vi "ErrorHandling.vi"() -> ()   [LabVIEW 2012]
uses:
  <vilib>/Utility/miscctls.llb/LVPointTypeDef.ctl
  Control and Global/Global_Variables.vi
  <vilib>/Utility/error.llb/DialogType.ctl
panel:
  out "Last Error/Warning":string
  out "Error Warning History":string[][](table)
  in  "Clear Hist":bool
  in  "Show Internal Errors":bool
  out "H2 Detected":bool
  out "H2":bool
  out "N2":bool
  out "Em Stop 2":bool
  out "Em Stop Relay":bool
  out "H2 CO":bool
  out "O2":bool
  out "Air":bool
  out "USV: No 230V":bool
  out "Watch Dog":bool
  out "H2 100W":bool
  out "N2 100W":bool
  out "H2 CO 100W":bool
  out "O2 100W":bool
  out "Air 100W":bool
  out "New MesErr file to load 1kW":bool
  in  "More/Less":bool
  in  "Em Stop":bool
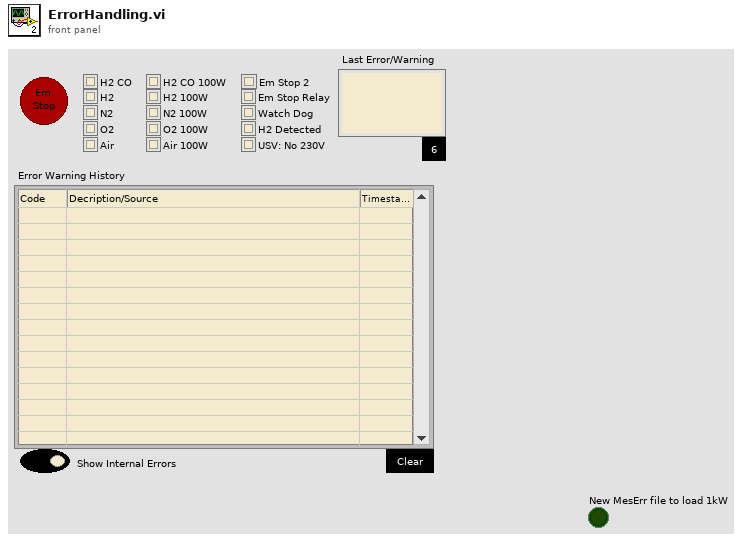
[diagram p1: front panel]
types:
  T1 = typedef "LVPointTypeDef.ctl" = cluster{"Horizontal":i16, "Vertical":i16}
  T2 = cluster{"Em. Button pressed":bool, "Em. Relay In":bool, "H2 detected":bool, "Watch Dog In":bool, "P_H2 not OK (1)":bool, "P_H2 not OK (2)":bool, "P_N2 not OK (1)":bool, "P_N2 not OK (2)":bool, "P_H2CO not OK (1)":bool, "P_H2CO not OK (2)":bool, "P_O2 not OK (1)":bool, "P_O2 not OK (2)":bool, "P_Air not OK (1)":bool, "P_Air not OK (2)":bool, "I/O 14 MUX":bool, "I/O 15 MUX":bool, "I/O 5":bool, "EM Stop Relay Out":bool, "Watch Dog Out":bool, "USV: No ~230V":bool}
  T3 = cluster{"f1":bool, "f2":bool, "f2":bool, "f3":bool, "New MesErr file to load":bool, "New Command file to load":bool, "f6":bool, "f7":bool, "New MesErr file to load 100W":bool, "New Command file to load 100W":bool}
  T4 = cluster{"Internal Error 1kW":bool, "Test Error 1kW":bool, "Shut down test":bool, "Terminate programm":bool, "Set secure state":bool, "Test is running":bool, "Flush after Error 1kW":bool, "f07":bool, "f08":bool, "Command file created":bool, "f10":bool, "f11":bool, "f12":bool, "f13":bool, "Logging":bool, "Is Measuring Cell Imp.":bool, "Test is running 100W":bool, "Command file created 100W":bool, "Shut down test 100W":bool, "Logging 100W":bool, "Internal Error 100W":bool, "Test Error 100W":bool, "Internal Error":bool, "Set secure state 100W":bool, "Flush after Error 100W":bool, "Init_Dnet":bool, "Use Stopsequenz 1kW":bool, "Use Stopsequenz 100W":bool, "Do Stopsequenz 1kW":bool, "Do Stopsequenz 100W":bool}
  T5 = typedef "Semaphore RefNum" = refnum<k1>
  T6 = typedef "DialogType.ctl" = u16
  T7 = typedef "TB1kW_Controls.lvlib/Format_Error.ctl" = cluster{"Name":string, "Options":dbl[], "Last check at:":timestamp}
  T8 = typedef "TB1kW_Controls.lvlib/Test_Properties.ctl" = cluster{"Cell Properties":T9, "Time":T10, "Flow N2 to Ox [Nl/min]":dbl, "Flow N2 to Fuel [Nl/min]":dbl, "Flush time after test error [s]":dbl, "Used Gases":cluster{"H2":bool, "N2":bool, "Air":bool, "O2":bool, "CO H2":bool}, "Fuelcell Temp. [°C]":dbl, "CO mixing ratio in tank [ppm]":dbl, "Stoichiometry Fuel [-]":dbl, "N2 in Fuel [%]":dbl, "Stoichiometry Ox [-]":dbl, "CO in Fuel [ppm]":dbl, "Humidity Ox [%]":dbl, "Humidity Fuel [%]":dbl, "Making I/U Curve":bool, "Meas Cell Impedance":bool, "Imped. Meas Intervall [s]":u32, "Nr. of Comand-Files Rep.":u32, "Use PS1":bool, "Use PS2":bool, "Use cyrostat":bool, "Used Temp Sens":cluster{"Temp 0":bool, "Temp 1":bool, "Temp 2":bool, "Temp 3":bool, "Temp 4":bool, "Temp 5":bool, "Temp 6":bool, "Temp 7":bool}, "Adjust AIn":cluster{"Gain":dbl, "Zero":dbl, "Unit":string}[]}
  T9 = typedef "TB1kW_Controls.lvlib/Cell_Properties.ctl" = cluster{"Nr of cells [-]":u8, "Cell area [cm2]":dbl, "Min. stack voltage [V]":dbl, "Min. cell voltage [mV]":dbl, "Max. stack current [A]":dbl, "Max. Dcell voltage [mV]":dbl, "Last Cell on Pin":i8, "First Cell on Pin":i8}
  T10 = typedef "TB1kW_Controls.lvlib/Time.ctl" = cluster{"[hh:mm:ss]\n[DD/MM/YY]":timestamp, "Include date":bool, "Time used as":string, "[hh:mm:ss]":dbl}
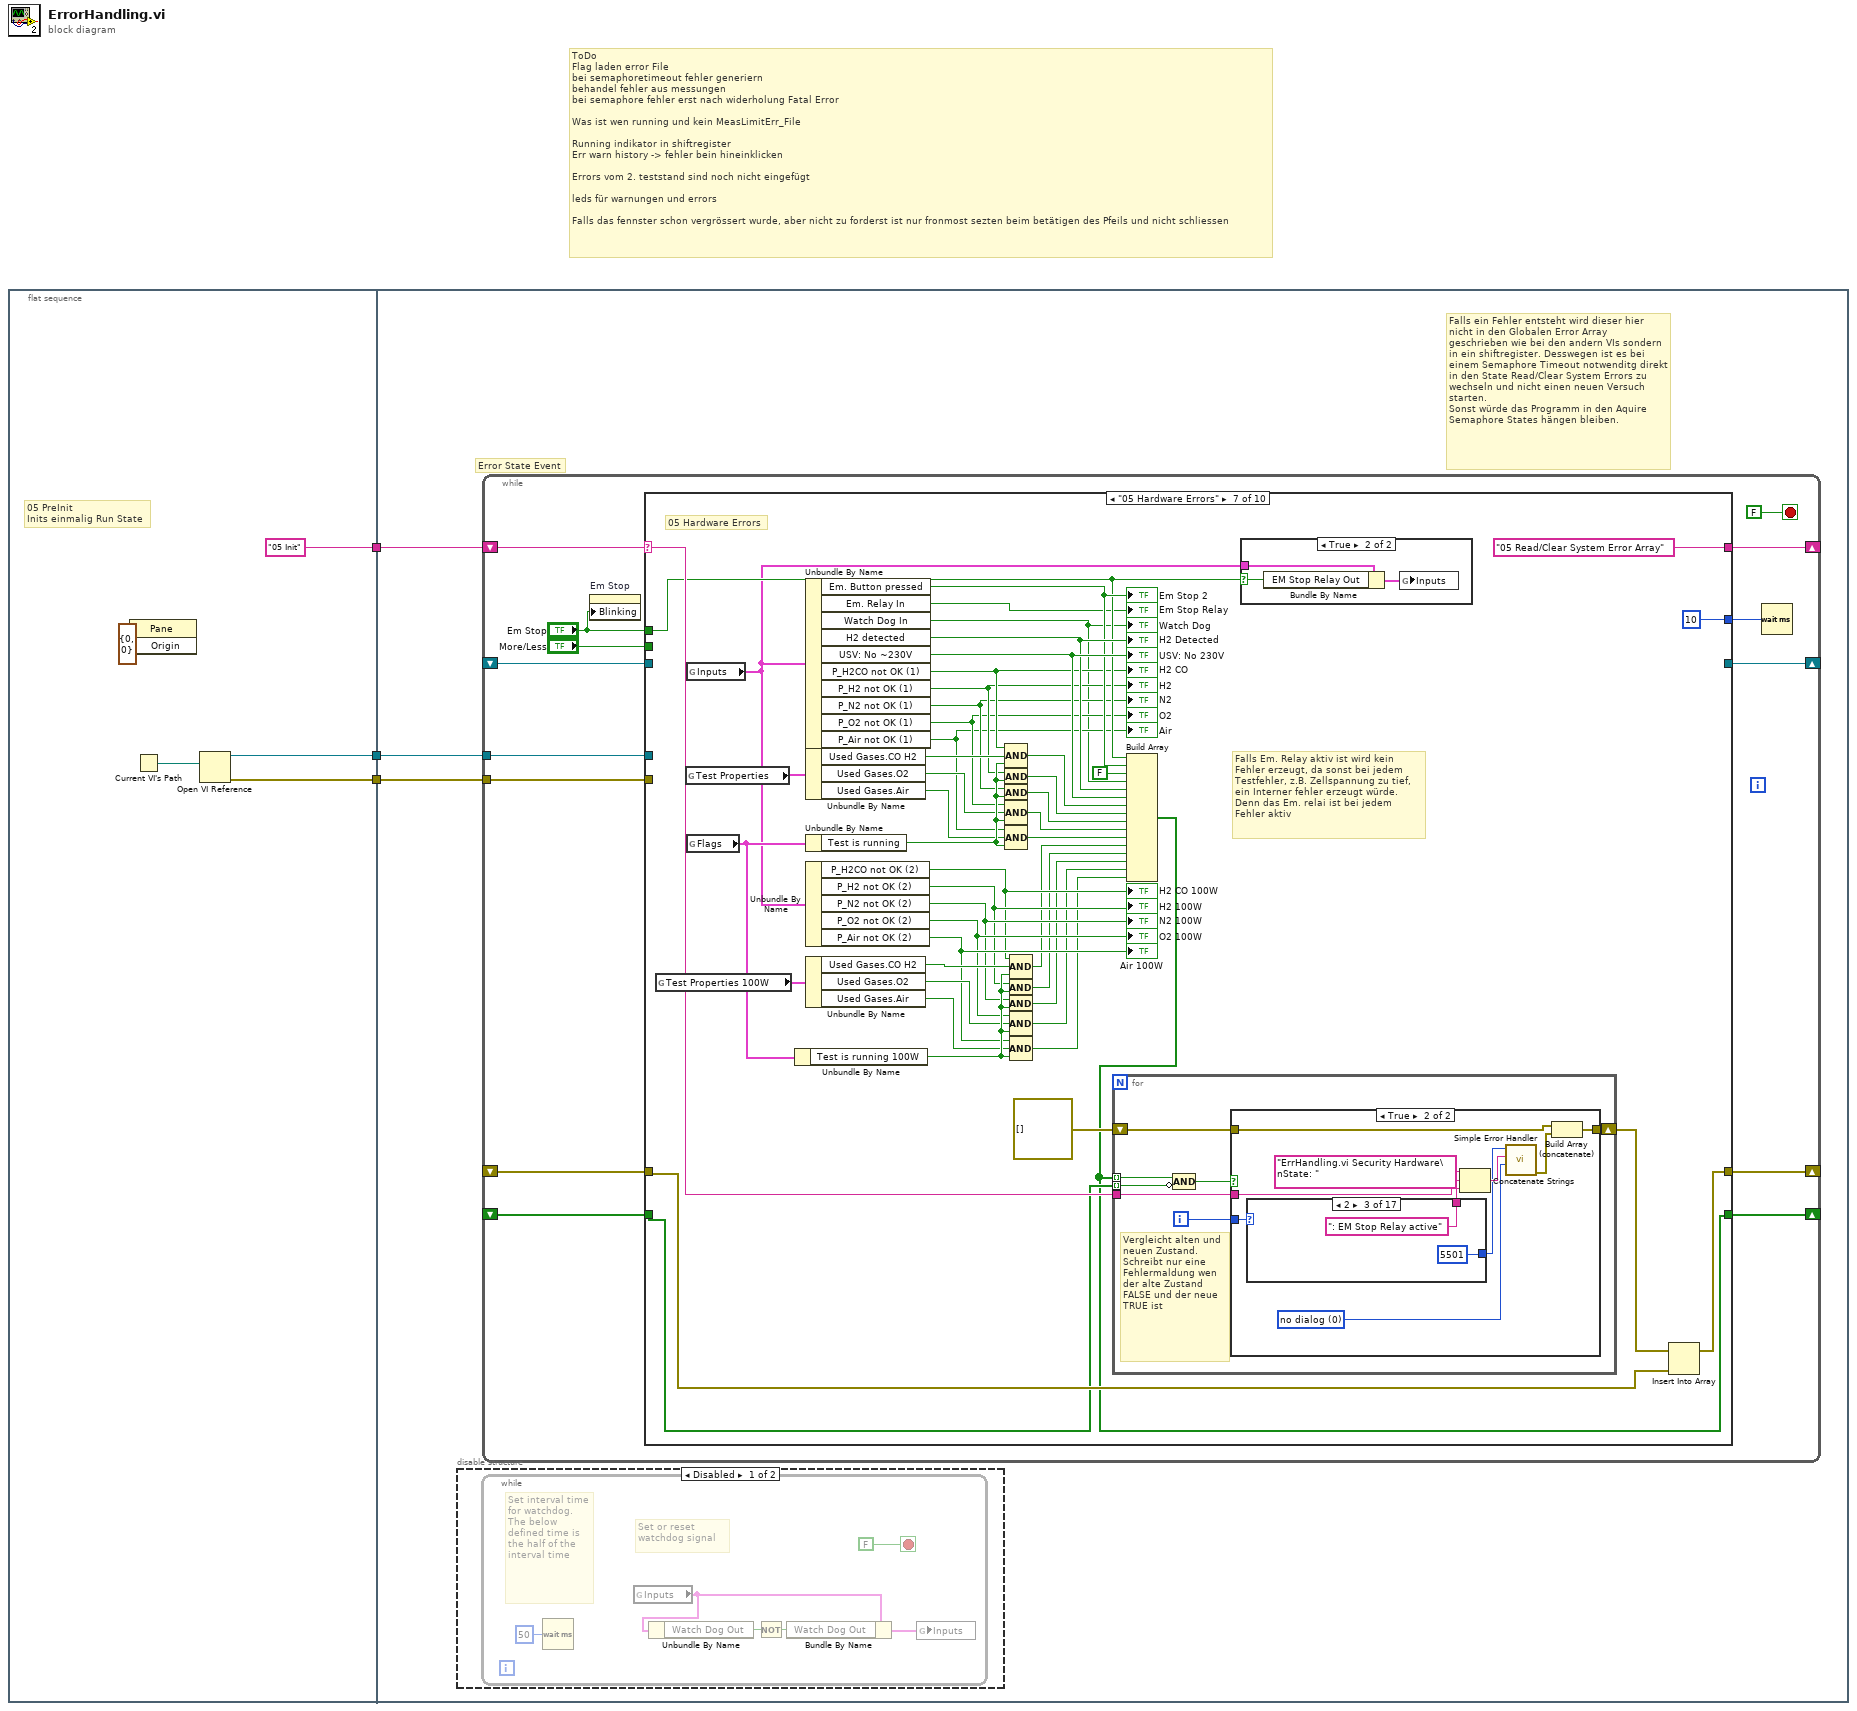
[diagram p0: block diagram]
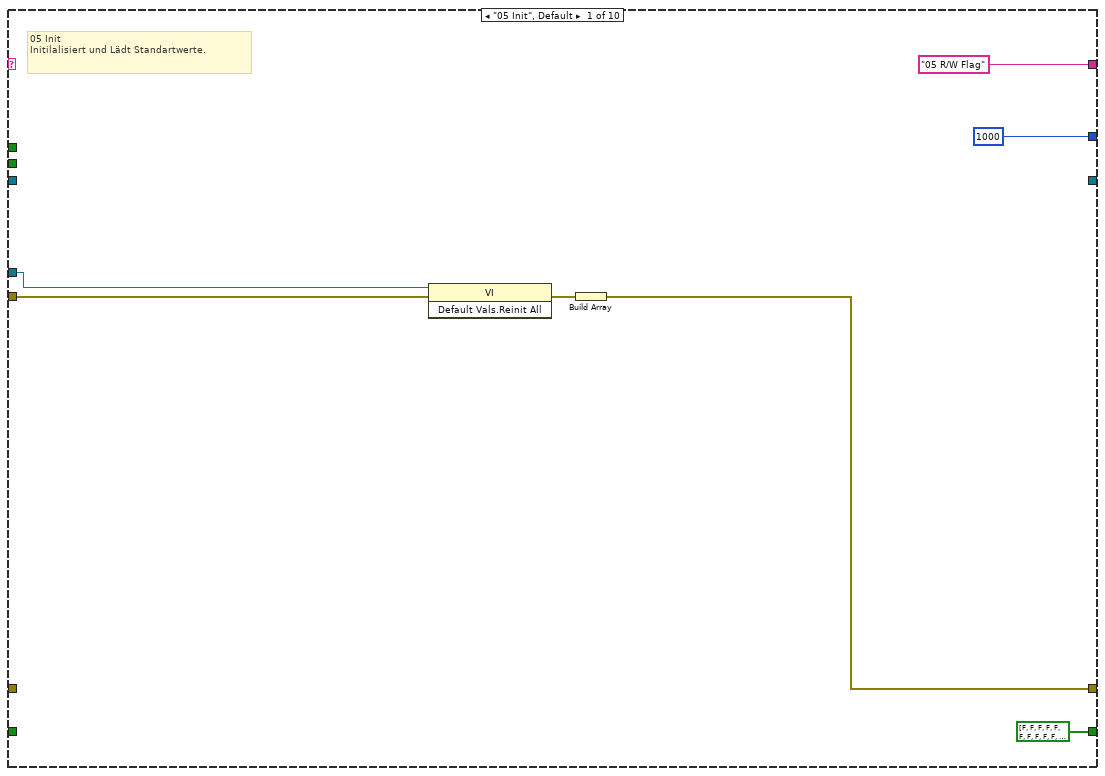
[diagram p3: hidden frame]
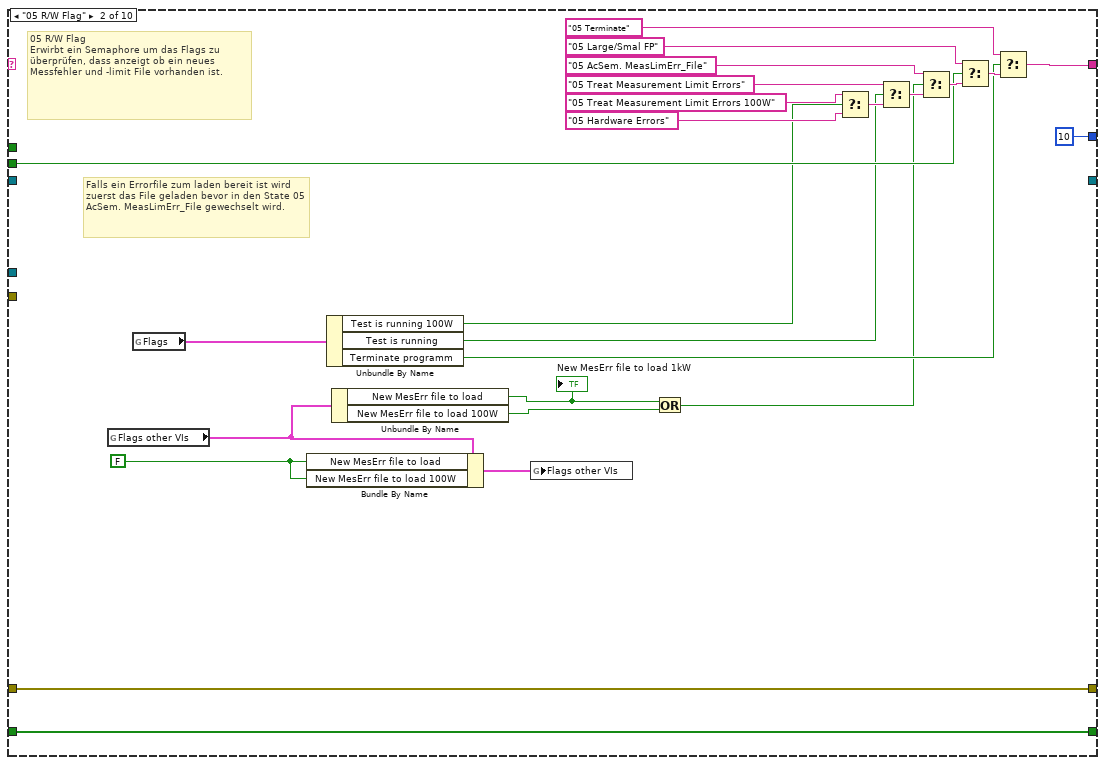
[diagram p4: hidden frame]
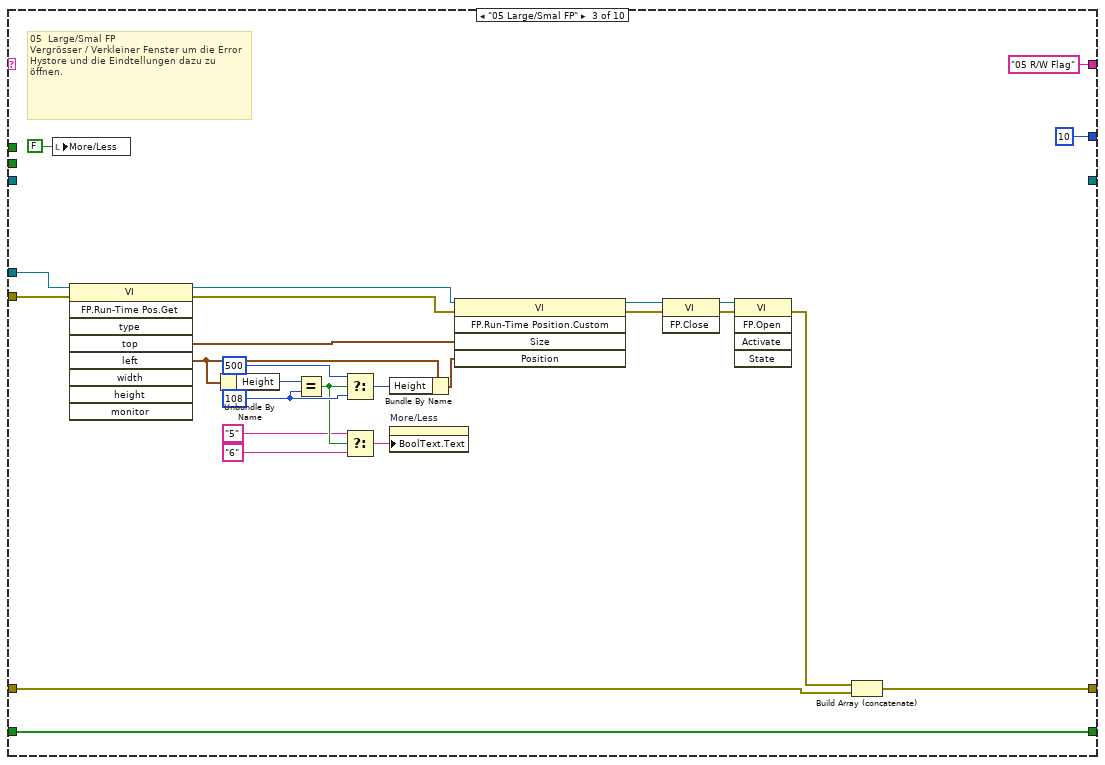
[diagram p5: hidden frame]
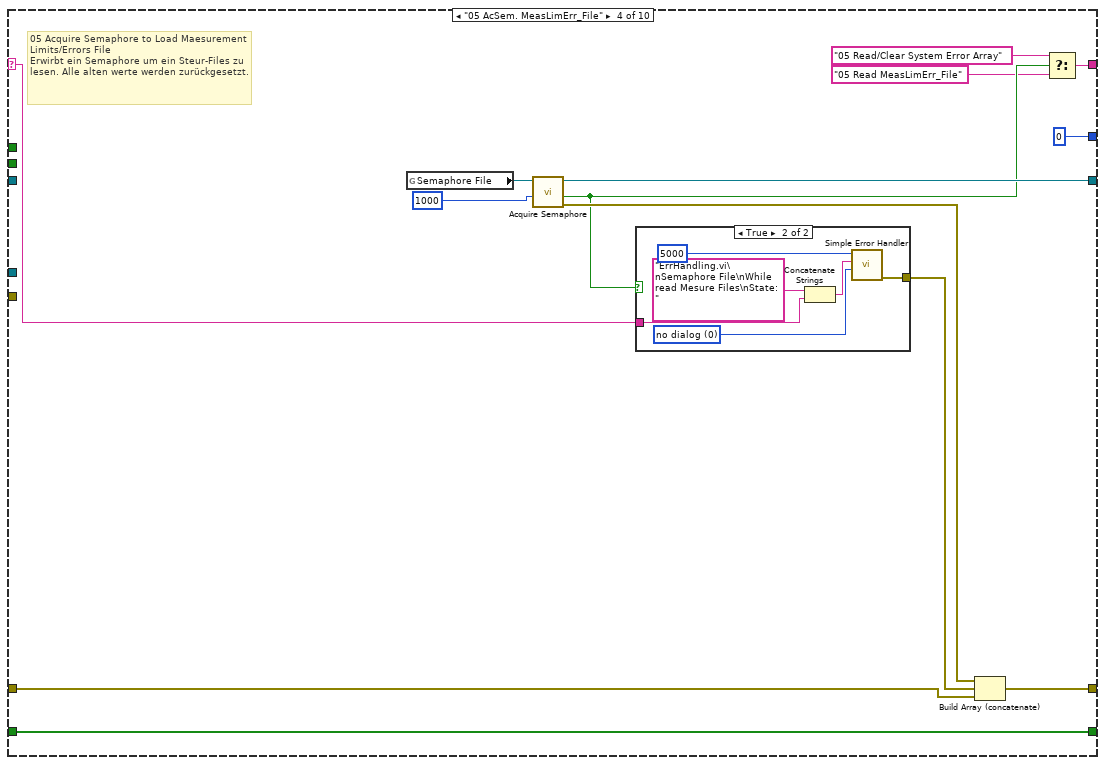
[diagram p6: hidden frame]
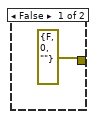
[diagram p7: hidden frame]
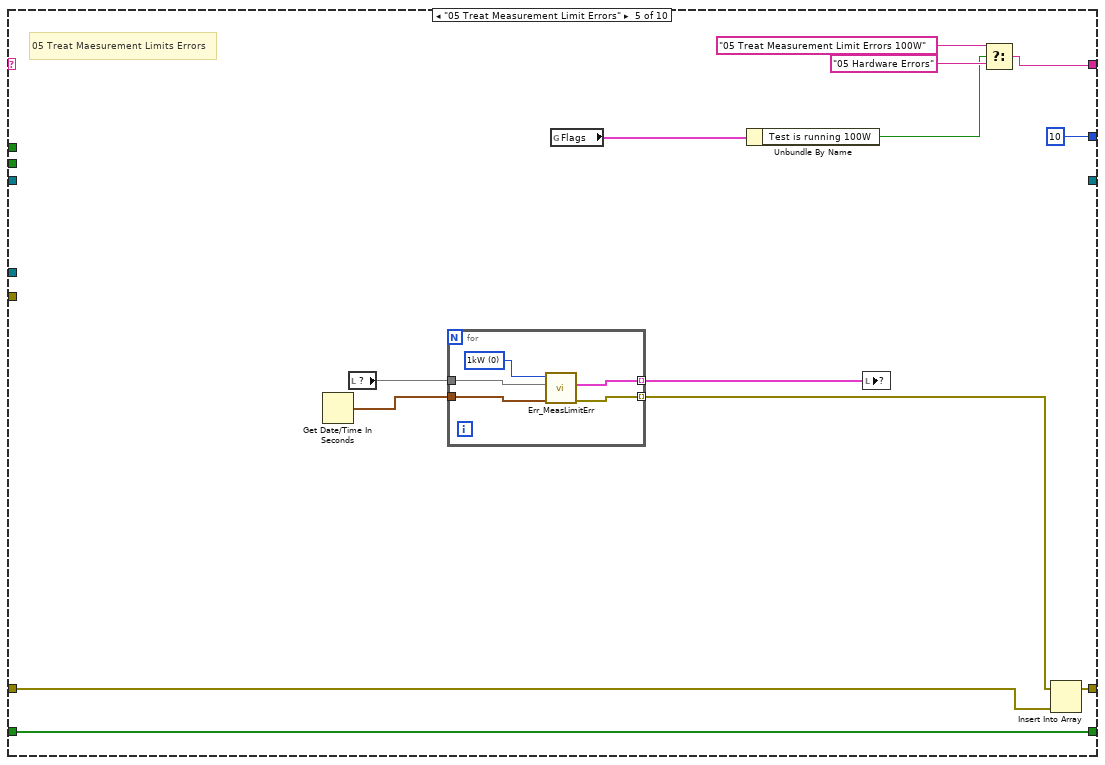
[diagram p8: hidden frame]
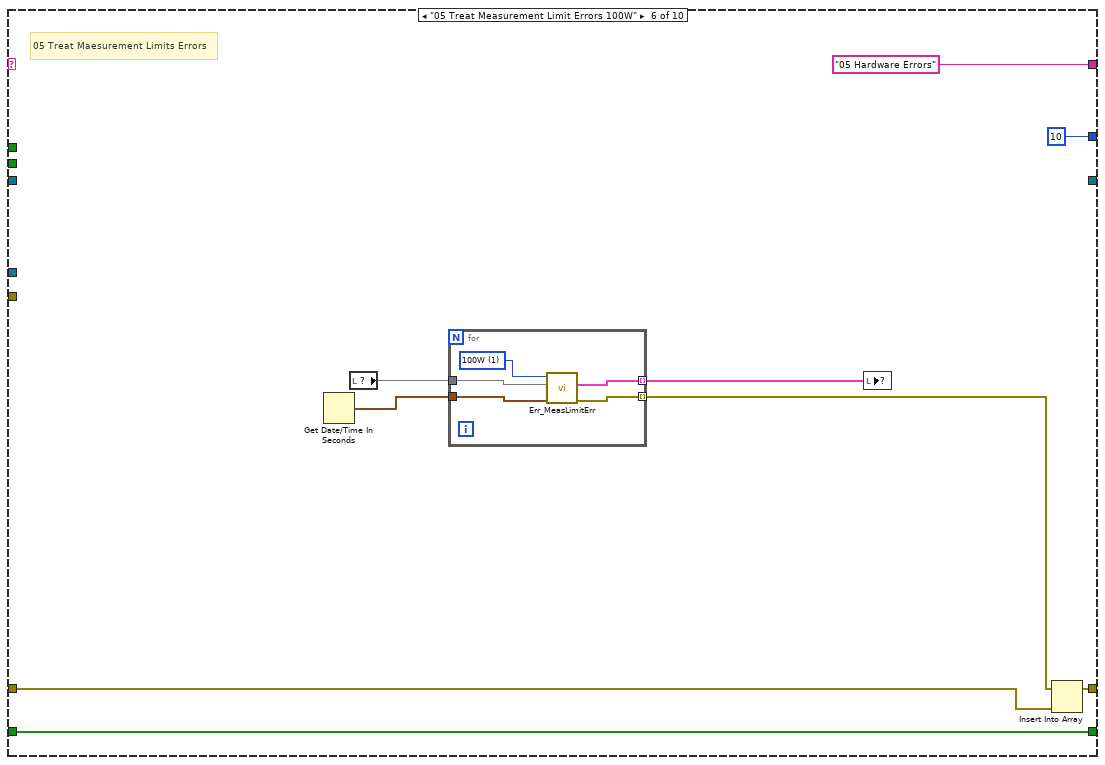
[diagram p9: hidden frame]
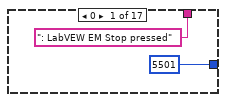
[diagram p12: hidden frame]
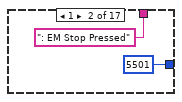
[diagram p13: hidden frame]
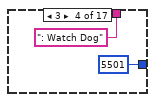
[diagram p14: hidden frame]
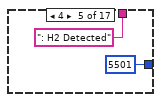
[diagram p15: hidden frame]
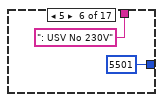
[diagram p16: hidden frame]
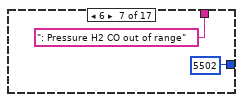
[diagram p17: hidden frame]
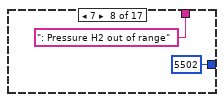
[diagram p18: hidden frame]
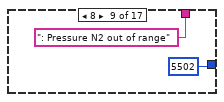
[diagram p19: hidden frame]
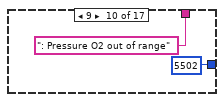
[diagram p20: hidden frame]
diagram:
  # "ToDo\nFlag laden error File\nbei semaphoretimeout fehler generiern\nbehandel fehler aus messungen\nbei semaphore fehler erst nach widerholung Fatal Error\n\nWas ist wen running und kein MeasLimitErr_File\n\nRunning indikator in shiftregister\nErr warn history -> fehler bein hineinklicken\n\nErrors vom 2. teststand sind noch nicht eingefügt\n\nleds für warnungen und errors\n\nFalls das fennster schon vergrössert wurde, aber nicht zu forderst ist nur fronmost sezten beim betätigen des Pfeils und nicht schliessen"
  n1 = flat-sequence {
    tunnel: [w8] -> w3
    tunnel: [w7] -> w2
    tunnel: ["05 Init" ("name or relative path")] -> w1
    tunnel: w3 -> [w11]
    tunnel: w2 -> [w10]
    tunnel: w1 -> [w9]
    frame #0 {
      # "05 PreInit\nInits einmalig Run State"
      n2 = property on="Property Node" class="Pane"("Origin"=T1 {"Horizontal"=0, "Vertical"=0}) -> ()  [unwired: 2 in, 2 out]
      n3 = Current VI's Path() -> (path=w6:path)
      n4 = Open VI Reference(vi path=w6) -> (vi reference=w8:refnum<vi>, error out=w7:errorcluster)  [unwired: 2 in, 3 out]
    }
    frame #1 {
      # "Falls ein Fehler entsteht wird dieser hier nicht in den Globalen Error Array geschrieben wie bei den andern VIs sondern in ein shiftregister. Desswegen ist es bei einem Semaphore Timeout notwenditg direkt in den State Read/Clear System Errors zu wechseln und nicht einen neuen Versuch starten.\nSonst würde das Programm in den Aquire Semaphore States hängen bleiben."
      # "Error State Event"
      n5 = disable-structure shown="Disabled" {
        frame Disabled {
          n6 = while {
            stop <- FALSE stop-if-true
            # "Set interval time for watchdog. The below defined time is the half of the interval time"
            # "Set or reset watchdog signal"
            n7 = Wait (ms)(milliseconds to wait=u32 50 ("Zu wartende ms")) -> ()  [unwired: 1 out]
            n8 = global read "Global_Variables.vi" "Inputs"() -> (w13:T2)
            n9 = Unbundle By Name(w13) -> ("Watch Dog Out"=w15:bool)
            n10 = Not(x=w15) -> (.not. x?=w16:bool)
            n11 = Bundle By Name(cluster=w13, "Watch Dog Out"=w16) -> (w14:T2)
            n12 = global write "Global_Variables.vi" "Inputs"(w14) -> ()
          }
        }
        frame Enabled {
        }
      }
      n13 = while {
        shift-right: [w24] -> _
        shift-left: w9 -> [w22]
        shift-right: [w29] -> _
        shift-left: _ -> [w28]
        tunnel: w11 -> [w27]
        tunnel: w10 -> [w26]
        shift-right: [w30] -> _
        shift-left: _ -> [w25]
        shift-right: [w20] -> _
        shift-left: _ -> [w19]
        stop <- FALSE stop-if-true
        n14 = property on="Em Stop" class="Bool (strict)"("Blinking"="Em Stop") -> ()  [unwired: 2 in, 2 out]
        n15 = case shown="\"05 Hardware Errors\"" w22 {
          selector: w22 -> [_ _ _ w97 _ _ w188 _ _ _]
          tunnel: ["05 R/W Flag" w50 "05 R/W Flag" w103 w111 "05 Hardware Errors" "05 Read/Clear System Error Array" "05 Treat All Errors" "05 R/W Flag" "05 Terminate"] -> w24
          tunnel: [u32 1000 ("milliseconds to wait") u32 10 ("milliseconds to wait") u32 10 ("milliseconds to wait") u32 0 ("milliseconds to wait") u32 10 ("milliseconds to wait") u32 10 ("milliseconds to wait") u32 10 ("milliseconds to wait") u32 10 ("milliseconds to wait") u32 10 ("milliseconds to wait") u32 10 ("milliseconds to wait")] -> w23
          tunnel: w28 -> [_ _ _ _ _ _ _ _ _ _]
          tunnel: w27 -> [w35 _ w80 _ _ _ _ _ _ w338]
          tunnel: w26 -> [w36 _ w79 _ _ _ _ _ _ w337]
          tunnel: [_ _ _ w96 _ _ _ _ _ _] -> w29
          tunnel: [w34 w61 w82 w93 w118 w132 w161 w248 errorcluster[] [] w334] -> w30
          tunnel: w25 -> [_ w61 w83 w94 w119 w131 w163 w249 w260 w333]
          tunnel: "More/Less" -> [_ w54 _ _ _ _ _ _ _ _]
          tunnel: "Em Stop" -> [_ _ _ _ _ _ w175 _ _ _]
          tunnel: [bool[] [FALSE, FALSE, FALSE, FALSE, FALSE, FALSE, FALSE, FALSE, FALSE, FALSE, FALSE, FALSE, FALSE, FALSE, FALSE, FALSE, FALSE, FALSE, FALSE, FALSE, FALSE] w52 w64 w90 w116 w133 w143 w246 w257 w331] -> w20
          tunnel: w19 -> [_ w52 w64 w90 w116 w133 w162 w246 w257 w331]
          frame "05 Init", Default {
            # "05 Init\nInitilalisiert und Lädt Standartwerte."
            n16 = invoke class="VI" method="Default Vals.Reinit All"(reference=w35, error in=w36) -> (error out=w37:errorcluster)  [unwired: 1 in, 2 out]
            n17 = Build Array(w37) -> (w34:errorcluster[])
          }
          frame "05 R/W Flag" {
            w44 = FALSE ("Measurement error file created")
            # "Falls ein Errorfile zum laden bereit ist wird zuerst das File geladen bevor in den State 05 AcSem. MeasLimErr_File gewechselt wird."
            # "05 R/W Flag\nErwirbt ein Semaphore um das Flags zu überprüfen, dass anzeigt ob ein neues Messfehler und -limit File vorhanden ist."
            n18 = global read "Global_Variables.vi" "Flags other VIs"() -> (w59:T3)
            n19 = global read "Global_Variables.vi" "Flags"() -> (w60:T4)
            n20 = Bundle By Name(cluster=w59, "New MesErr file to load"=w44, "New MesErr file to load 100W"=w44) -> (w58:T3)
            n21 = Unbundle By Name(w60) -> ("Test is running 100W"=w40:bool, "Test is running"=w39:bool, "Terminate programm"=w48:bool)
            n22 = Unbundle By Name(w59) -> ("New MesErr file to load"=w47:bool, "New MesErr file to load 100W"=w46:bool)
            "New MesErr file to load 1kW" <- w47
            n23 = global write "Global_Variables.vi" "Flags other VIs"(w58) -> ()
            n24 = Or(x=w47, y=w46) -> (x .or. y?=w45:bool)
            n25 = Select(t="05 Treat Measurement Limit Errors 100W", s=w40, f="05 Hardware Errors") -> (s? t:f=w43:string)
            n26 = Select(t="05 Treat Measurement Limit Errors", s=w39, f=w43) -> (s? t:f=w62:string)
            n27 = Select(t="05 AcSem. MeasLimErr_File", s=w45, f=w62) -> (s? t:f=w55:string)
            n28 = Select(t="05 Large/Smal FP", s=w54, f=w55) -> (s? t:f=w49:string)
            n29 = Select(t="05 Terminate", s=w48, f=w49) -> (s? t:f=w50:string)
          }
          frame "05 Large/Smal FP" {
            w86 = i16 108 ("y")
            # "05  Large/Smal FP\nVergrösser / Verkleiner Fenster um die Error Hystore und die Eindtellungen dazu zu öffnen."
            n30 = local write "More/Less"(FALSE ("More/Less")) -> ()
            n31 = invoke class="VI" method="FP.Run-Time Pos.Get"(reference=w80, error in=w79) -> (reference out=w77:refnum<vi>, error out=w76:errorcluster, "top"=w74:cluster{"Top":i16, "Left":i16}, "left"=w78:cluster{"Height":i16, "Width":i16})  [unwired: 7 in, 5 out]
            n32 = Unbundle By Name(w78) -> ("Height"=w87:i16)
            n33 = Equal?(x=w87, y=w86) -> (x = y?=w68:bool)
            n34 = Select(t=i16 500 ("y"), s=w68, f=w86) -> (s? t:f=w84:i16)
            n35 = Select(t="5", s=w68, f="6") -> (s? t:f=w65:string)
            n36 = Bundle By Name(cluster=w78, "Height"=w84) -> (w75:cluster{"Height":i16, "Width":i16})
            n37 = property on="More/Less" class="Bool (strict)"("BoolText.Text"=w65) -> ()  [unwired: 2 in, 2 out]
            n38 = invoke class="VI" method="FP.Run-Time Position.Custom"(reference=w77, error in=w76, "Size"=w74, "Position"=w75) -> (reference out=w72:refnum<vi>, error out=w71:errorcluster)  [unwired: 1 in, 3 out]
            n39 = invoke class="VI" method="FP.Close"(reference=w72, error in=w71) -> (reference out=w69:refnum<vi>, error out=w70:errorcluster)  [unwired: 1 in, 1 out]
            n40 = invoke class="VI" method="FP.Open"(reference=w69, error in=w70) -> (error out=w73:errorcluster)  [unwired: 3 in, 4 out]
            n41 = Build Array (concatenate)(w73, w83) -> (w82:errorcluster[])
          }
          frame "05 AcSem. MeasLimErr_File" {
            # "05 Acquire Semaphore to Load Maesurement Limits/Errors File\nErwirbt ein Semaphore um ein Steur-Files zu lesen. Alle alten werte werden zurückgesetzt."
            n42 = global read "Global_Variables.vi" "Semaphore File"() -> (w100:T5)
            n43 = call <vilib>:"Acquire Semaphore.vi"("ms timeout (-1)"=1000, "semaphore"=w100) -> ("error out"=w99:errorcluster, "timed out"=w95:bool, "semaphore out"=w96:T5)  [unwired: 1 in, 2 out]
            n44 = case shown="True" w95 {
              tunnel: [errorcluster {"status"=FALSE, "code"=0, "source"=""} ("error out") w108] -> w98
              tunnel: w97 -> [_ w105]
              frame False {
              }
              frame True {
                w109 = T6 0 items=["no dialog", "OK message", "continue or stop message", "OK message + warnings", "continue/stop + warnings"] ("type of dialog (OK msg:1)")
                n45 = Concatenate Strings("ErrHandling.vi\nSemaphore File\nWhile read Mesure Files\nState: " ("error source (\" \")"), w105) -> (w106:string)
                n46 = call <vilib>:"Simple Error Handler.vi"("error code (no error:0)"=5000, "error source (\" \")"=w106, "type of dialog (OK msg:1)"=w109) -> ("error out"=w108:errorcluster)  [unwired: 1 in, 5 out]
              }
            }
            n47 = Build Array (concatenate)(w99, w98, w94) -> (w93:errorcluster[])
            n48 = Select(t="05 Read/Clear System Error Array", s=w95, f="05 Read MeasLimErr_File") -> (s? t:f=w103:string)
          }
          frame "05 Treat Measurement Limit Errors" {
            # "05 Treat Maesurement Limits Errors"
            n49 = Get Date/Time In Seconds() -> (seconds since 1Jan1904=w117:timestamp)
            n50 = local read item#-1() -> (w122)
            n51 = for {
              tunnel: w122 -> [w126]
              tunnel: [w128] -> w121 mode=indexing
              tunnel: [w127] -> w120 mode=indexing
              tunnel: w117 -> [w125]
              w124 = u8 0 items=["1kW", "100W"] ("Testbench")
              n52 = call "Err_MeasLimitErr.vi"("Current time"=w125, "Measurement Error Limit In"=w126, "Testbench"=w124) -> ("Error out"=w127:errorcluster, "Measurement Error Limit Out"=w128:T7)  [unwired: 3 out]
            }
            n53 = global read "Global_Variables.vi" "Flags"() -> (w115:T4)
            n54 = Unbundle By Name(w115) -> ("Test is running 100W"=w112:bool)
            n55 = local write item#-1(w121) -> ()
            n56 = Select(t="05 Treat Measurement Limit Errors 100W", s=w112, f="05 Hardware Errors") -> (s? t:f=w111:string)
            n57 = Insert Into Array(array=w120, new element=w119) -> (w118:errorcluster[])  [unwired: 1 in]
          }
          frame "05 Treat Measurement Limit Errors 100W" {
            # "05 Treat Maesurement Limits Errors"
            n58 = Get Date/Time In Seconds() -> (seconds since 1Jan1904=w134:timestamp)
            n59 = local read item#-1() -> (w137)
            n60 = for {
              tunnel: w137 -> [w140]
              tunnel: [w142] -> w136 mode=indexing
              tunnel: [w141] -> w135 mode=indexing
              tunnel: w134 -> [w139]
              w138 = u8 1 items=["1kW", "100W"] ("Testbench")
              n61 = call "Err_MeasLimitErr.vi"("Current time"=w139, "Measurement Error Limit In"=w140, "Testbench"=w138) -> ("Error out"=w141:errorcluster, "Measurement Error Limit Out"=w142:T7)  [unwired: 3 out]
            }
            n62 = local write item#-1(w136) -> ()
            n63 = Insert Into Array(array=w135, new element=w131) -> (w132:errorcluster[])  [unwired: 1 in]
          }
          frame "05 Hardware Errors" {
            # "Falls Em. Relay aktiv ist wird kein Fehler erzeugt, da sonst bei jedem Testfehler, z.B. Zellspannung zu tief, ein Interner fehler erzeugt würde. Denn das Em. relai ist bei jedem Fehler aktiv"
            # "05 Hardware Errors"
            n64 = global read "Global_Variables.vi" "Test Properties 100W"() -> (w160:T8)
            n65 = global read "Global_Variables.vi" "Test Properties"() -> (w183:T8)
            n66 = global read "Global_Variables.vi" "Inputs"() -> (w144:T2)
            n67 = global read "Global_Variables.vi" "Flags"() -> (w155:T4)
            n68 = Unbundle By Name(w155) -> ("Test is running 100W"=w158:bool)
            n69 = Unbundle By Name(w144) -> ("Em. Button pressed"=w176:bool, "Em. Relay In"=→"Em Stop Relay":bool, "Watch Dog In"=w169:bool, "H2 detected"=w177:bool, "USV: No ~230V"=w178:bool, "P_H2CO not OK (1)"=w174:bool, "P_H2 not OK (1)"=w173:bool, "P_N2 not OK (1)"=w172:bool, "P_O2 not OK (1)"=w171:bool, "P_Air not OK (1)"=w170:bool)
            "H2 Detected" <- w177
            "H2" <- w173
            "N2" <- w172
            "Em Stop 2" <- w176
            "H2 CO" <- w174
            "O2" <- w171
            "Air" <- w170
            "USV: No 230V" <- w178
            "Watch Dog" <- w169
            n70 = Unbundle By Name(w183) -> ("Used Gases.CO H2"=w182:bool, "Used Gases.O2"=w180:bool, "Used Gases.Air"=w179:bool)
            n71 = Unbundle By Name(w155) -> ("Test is running"=w181:bool)
            n72 = Unbundle By Name(w144) -> ("P_H2CO not OK (2)"=w150:bool, "P_H2 not OK (2)"=w151:bool, "P_N2 not OK (2)"=w152:bool, "P_O2 not OK (2)"=w153:bool, "P_Air not OK (2)"=w154:bool)
            "H2 100W" <- w151
            "N2 100W" <- w152
            "H2 CO 100W" <- w150
            "O2 100W" <- w153
            "Air 100W" <- w154
            n73 = Unbundle By Name(w160) -> ("Used Gases.CO H2"=w159:bool, "Used Gases.O2"=w157:bool, "Used Gases.Air"=w156:bool)
            n74 = And(x=w173, y=w181) -> (x .and. y?=w164:bool)
            n75 = And(x=w172, y=w181) -> (x .and. y?=w166:bool)
            n76 = Compound Arithmetic op=AND(w174, w182, w181) -> (w165:bool)
            n77 = Compound Arithmetic op=AND(w171, w180, w181) -> (w185:bool)
            n78 = Compound Arithmetic op=AND(w170, w179, w181) -> (w184:bool)
            n79 = And(x=w151, y=w158) -> (x .and. y?=w148:bool)
            n80 = And(x=w152, y=w158) -> (x .and. y?=w147:bool)
            n81 = Compound Arithmetic op=AND(w150, w159, w158) -> (w149:bool)
            n82 = Compound Arithmetic op=AND(w153, w157, w158) -> (w146:bool)
            n83 = Compound Arithmetic op=AND(w154, w156, w158) -> (w145:bool)
            n84 = Build Array(w175, w176, FALSE ("Element"), w169, w177, w178, w165, w164, w166, w185, w184, w149, w148, w147, w146, w145) -> (w143:bool[])
            n85 = for {
              tunnel: w143 -> [w199] mode=indexing
              tunnel: w162 -> [w200] mode=indexing
              shift-right: [w198] -> w186
              shift-left: errorcluster[] [] -> [w197]
              tunnel: w188 -> [w194]
              i -> [w195]
              # "Vergleicht alten und neuen Zustand.\nSchreibt nur eine Fehlermaldung wen der alte Zustand FALSE und der neue TRUE ist"
              n86 = Compound Arithmetic op=AND(w199, invert w200) -> (w196:bool)
              n87 = case shown="True" w196 {
                tunnel: [w201 w205] -> w198
                tunnel: w197 -> [w201 w207]
                tunnel: w195 -> [_ w204]
                tunnel: w194 -> [_ w208]
                frame False {
                }
                frame True {
                  w211 = T6 0 items=["no dialog", "OK message", "continue or stop message", "OK message + warnings", "continue/stop + warnings"] ("type of dialog (OK msg:1)")
                  n88 = case shown="2" w204 {
                    tunnel: [": LabVEW EM Stop pressed" ("error source (\" \")") ": EM Stop Pressed" ("error source (\" \")") ": EM Stop Relay active" ("error source (\" \")") ": Watch Dog" ("error source (\" \")") ": H2 Detected" ("error source (\" \")") ": USV No 230V" ("error source (\" \")") ": Pressure H2 CO out of range" ("error source (\" \")") ": Pressure H2 out of range" ("error source (\" \")") ": Pressure N2 out of range" ("error source (\" \")") ": Pressure O2 out of range" ("error source (\" \")") ": Pressure Air out of range" ("error source (\" \")") ": Pressure H2 CO 100W out of range" ("error source (\" \")") ": Pressure H2 100W out of range" ("error source (\" \")") ": Pressure N2 100W out of range" ("error source (\" \")") ": Pressure O2 100W out of range" ("error source (\" \")") ": Pressure Air 100W out of range" ("error source (\" \")") ": Input not known " ("error source (\" \")")] -> w203
                    tunnel: [5501 ("error code (no error:0)") 5501 ("error code (no error:0)") 5501 ("error code (no error:0)") 5501 ("error code (no error:0)") 5501 ("error code (no error:0)") 5501 ("error code (no error:0)") 5502 ("error code (no error:0)") 5502 ("error code (no error:0)") 5502 ("error code (no error:0)") 5502 ("error code (no error:0)") 5502 ("error code (no error:0)") 5503 ("error code (no error:0)") 5503 ("error code (no error:0)") 5503 ("error code (no error:0)") 5503 ("error code (no error:0)") 5503 ("error code (no error:0)") 5501 ("error code (no error:0)")] -> w202
                    frame 0 {
                    }
                    frame 1 {
                    }
                    frame 2 {
                    }
                    frame 3 {
                    }
                    frame 4 {
                    }
                    frame 5 {
                    }
                    frame 6 {
                    }
                    frame 7 {
                    }
                    frame 8 {
                    }
                    frame 9 {
                    }
                    frame 10 {
                    }
                    frame 11 {
                    }
                    frame 12 {
                    }
                    frame 13 {
                    }
                    frame 14 {
                    }
                    frame 15 {
                    }
                    frame 21, Default {
                    }
                  }
                  n89 = Concatenate Strings("ErrHandling.vi Security Hardware\nState: " ("error source (\" \")"), w208, w203) -> (w209:string)
                  n90 = call <vilib>:"Simple Error Handler.vi"("error code (no error:0)"=w202, "error source (\" \")"=w209, "type of dialog (OK msg:1)"=w211) -> ("error out"=w206:errorcluster)  [unwired: 1 in, 5 out]
                  n91 = Build Array (concatenate)(w207, w206) -> (w205:errorcluster[])
                }
              }
            }
            n92 = case shown="True" w175 {
              selector: w175 -> [_ w191]
              tunnel: w144 -> [_ w192]
              frame False {
              }
              frame True {
                n93 = Bundle By Name(cluster=w192, "EM Stop Relay Out"=w191) -> (w193:T2)
                n94 = global write "Global_Variables.vi" "Inputs"(w193) -> ()
              }
            }
            n95 = Insert Into Array(array=w186, new element=w163) -> (w161:errorcluster[])  [unwired: 1 in]
          }
          frame "05 Read/Clear System Error Array" {
            # "05 Read and Clear System Error Array\nLiest den System Error Array aus und fügt ihn mit den anderen Fehlern zusammen um diese danach zu beareuiten. Der System Error Array wird danach gelöscht"
            n96 = flat-sequence {
              tunnel: [w252] -> w250
              frame #0 {
                n97 = global read "Global_Variables.vi" "Errors"() -> (w252:errorcluster[])
              }
              frame #1 {
                n98 = global write "Global_Variables.vi" "Errors"(errorcluster[] []) -> ()
              }
            }
            n99 = Insert Into Array(array=w250, new element=w249) -> (w248:errorcluster[])  [unwired: 1 in]
          }
          frame "05 Treat All Errors" {
            # "05 Treat All Errors\nHier werden alle Fehler behandelt\nund die im gesamten System auftretn"
            n100 = case shown="True" "Clear Hist" {
              tunnel: [w264 string[][] []] -> w255
              frame False {
                n101 = local read "Error Warning History"() -> (w264:string[][])
              }
              frame True {
                n102 = local write "Last Error/Warning"("" ("Last Error/Warning")) -> ()
              }
            }
            n103 = Get Date/Time In Seconds() -> (seconds since 1Jan1904=w259:timestamp)
            n104 = for {
              tunnel: w260 -> [w272] mode=indexing
              tunnel: w259 -> [w271]
              shift-right: [w267] -> w258
              shift-left: w255 -> [w268]
              tunnel: "Show Internal Errors" -> [w270]
              n105 = Unbundle By Name(w272) -> ("code"=w273:i32)
              n106 = case shown="5501" w273 {
                tunnel: w272 -> [_ _ _ _ _ _ _ _ w313 w320 w325]
                tunnel: [_ TRUE ("Fatal Error") _ w301 w304 _ _ _ TRUE ("Fatal Error") TRUE ("Fatal Error") TRUE ("Fatal Error")] -> w269
                frame 0, Default {
                }
                frame -8501, -8500 {
                }
                frame 5000 {
                  # "Semaphore Time out"
                }
                frame 6000..6006 {
                  w301 = TRUE ("Fatal Error")
                  # "Test Errors"
                  n107 = global read "Global_Variables.vi" "Flags"() -> (w302:T4)
                  n108 = Bundle By Name(cluster=w302, "Test Error 1kW"=w301) -> (w303:T4)
                  n109 = global write "Global_Variables.vi" "Flags"(w303) -> ()
                }
                frame 6007..6013 {
                  w304 = TRUE ("Fatal Error")
                  # "Test Errors"
                  n110 = global read "Global_Variables.vi" "Flags"() -> (w306:T4)
                  n111 = Bundle By Name(cluster=w306, "Test Error 100W"=w304) -> (w305:T4)
                  n112 = global write "Global_Variables.vi" "Flags"(w305) -> ()
                }
                frame 5011 {
                  # "Unable to write Error"
                  n113 = global read "Global_Variables.vi" "Flags"() -> (w307:T4)
                  n114 = Bundle By Name(cluster=w307, "Internal Error 100W"=TRUE ("Fatal Error")) -> (w308:T4)
                  n115 = global write "Global_Variables.vi" "Flags"(w308) -> ()
                }
                frame 5010 {
                  # "Unable to write output"
                  n116 = global read "Global_Variables.vi" "Flags"() -> (w312:T4)
                  n117 = Bundle By Name(cluster=w312, "Internal Error 1kW"=TRUE ("Fatal Error")) -> (w311:T4)
                  n118 = global write "Global_Variables.vi" "Flags"(w311) -> ()
                }
                frame 5012 {
                }
                frame 5501 {
                  # "Security hardware error"
                  n119 = Unbundle By Name(w313) -> ()  [unwired: 2 out]
                  n120 = case shown="True" TRUE {
                    frame False {
                    }
                    frame True {
                      n121 = global read "Global_Variables.vi" "Flags"() -> (w318:T4)
                      n122 = Bundle By Name(cluster=w318, "Internal Error"=TRUE ("Fatal Error")) -> (w317:T4)
                      n123 = global write "Global_Variables.vi" "Flags"(w317) -> ()
                    }
                  }
                }
                frame 5502 {
                  # "Security hardware error"
                  n124 = Unbundle By Name(w320) -> ()  [unwired: 2 out]
                  n125 = case shown="True" TRUE {
                    frame False {
                    }
                    frame True {
                      n126 = global read "Global_Variables.vi" "Flags"() -> (w324:T4)
                      n127 = Bundle By Name(cluster=w324, "Internal Error 1kW"=TRUE ("Fatal Error")) -> (w323:T4)
                      n128 = global write "Global_Variables.vi" "Flags"(w323) -> ()
                    }
                  }
                }
                frame 5503 {
                  # "Security hardware error"
                  n129 = Unbundle By Name(w325) -> ()  [unwired: 2 out]
                  n130 = case shown="True" TRUE {
                    frame False {
                    }
                    frame True {
                      n131 = global read "Global_Variables.vi" "Flags"() -> (w330:T4)
                      n132 = Bundle By Name(cluster=w330, "Internal Error 100W"=TRUE ("Fatal Error")) -> (w329:T4)
                      n133 = global write "Global_Variables.vi" "Flags"(w329) -> ()
                    }
                  }
                }
              }
              n134 = case shown="Error" w272 {
                selector: w272 -> [_ w283]
                tunnel: w268 -> [w274 w280]
                tunnel: [w274 w279] -> w267
                tunnel: w271 -> [_ w282]
                tunnel: w270 -> [_ w277]
                tunnel: w269 -> [_ w276]
                frame No Error {
                }
                frame Error {
                  n135 = Unbundle By Name(w283) -> ("code"=w281:i32, "source"=w278:string)
                  n136 = Or(x=w276, y=w277) -> (x .or. y?=w275:bool)
                  n137 = case shown="True" w275 {
                    tunnel: w282 -> [_ w299]
                    tunnel: w281 -> [_ w297]
                    tunnel: w280 -> [w284 w296]
                    tunnel: [w284 w295] -> w279
                    tunnel: w278 -> [_ w287]
                    frame False {
                    }
                    frame True {
                      w289 = ": " ("String")
                      n138 = Get Date/Time String(date format (0)=enum16{"short", "long", "abbreviated"}."long", seconds (now)=w299, want seconds? (F)=TRUE) -> (date string=w292:string, time string=w291:string)
                      n139 = Number To Decimal String(number=w297) -> (decimal integer string=w290:string)  [unwired: 1 out]
                      n140 = Concatenate Strings(w291, "\r", w292) -> (w288:string)
                      n141 = Build Array(w290, w287, w288) -> (w285:string[])
                      n142 = Concatenate Strings(w290, w289, w287, w289, w288, w289) -> (→"Last Error/Warning":string)
                      n143 = Build Array (concatenate)(w285, w296) -> (w295:string[][])
                    }
                  }
                }
              }
            }
            "Error Warning History" <- w258
          }
          frame "05 Terminate" {
            # "(Wird nicht mehr ausgeführt)"
            # "05 Terminate"
            n144 = invoke class="VI" method="FP.Close"(reference=w338, error in=w337) -> (reference out=w335:refnum<vi>, error out=w336:errorcluster)  [unwired: 1 in, 1 out]
            n145 = invoke class="VI" method="Abort VI"(reference=w335, error in=w336) -> (error out=w339:errorcluster)  [unwired: 1 in, 2 out]
            n146 = Build Array (concatenate)(w339, w333) -> (w334:errorcluster[])
          }
        }
        n147 = Wait (ms)(milliseconds to wait=w23) -> ()  [unwired: 1 out]
      }
    }
  }
